vi "Get First 429 Tx Channel.vi"(8 "error in (no error)":errorcluster, 11 "Card Number":i32=2) -> (0 "error out":errorcluster, 2 "Channel Number":i32=32, 3 "Core Number":i32)   [LabVIEW 2019]
uses:
  <instrlib>/BTICardLib/Private/Initialize By Card Number and Core Number.vi
  <instrlib>/BTICardLib/BTICardLV.lvlib
  <instrlib>/BTI429Lib/BTI429LV.lvlib
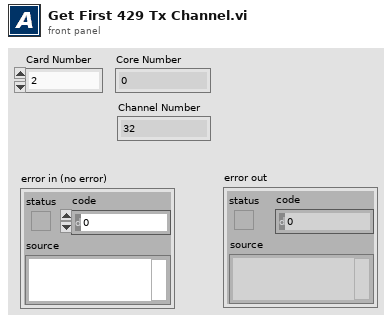
[diagram p1: front panel]
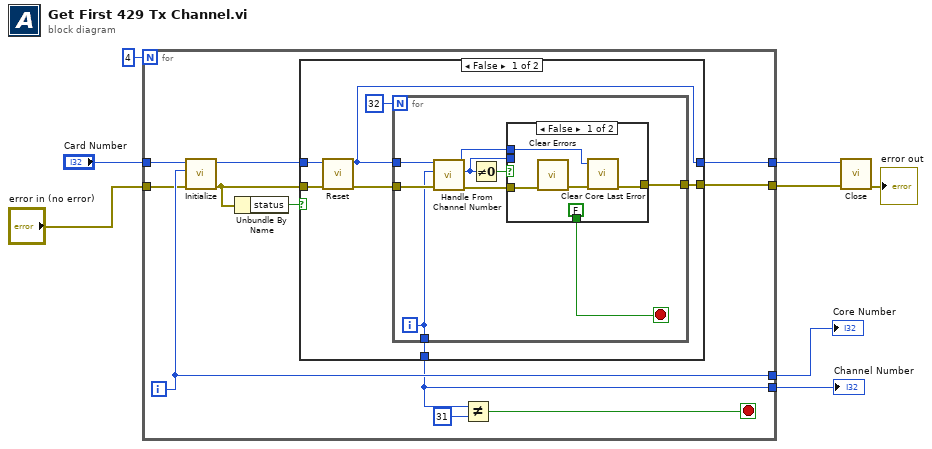
[diagram p0: block diagram]
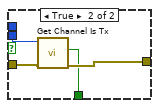
[diagram p2: hidden frame]
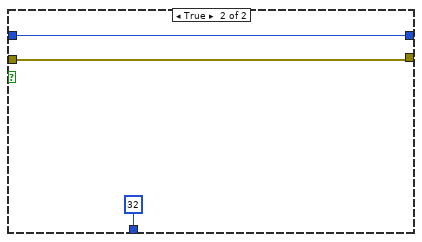
[diagram p3: hidden frame]
diagram:
  n1 = for {
    N: 4 -> [_]
    tunnel: "Card Number" -> [w19]
    tunnel: [w15] -> w6
    tunnel: [w12] -> w5
    tunnel: [w11] -> w4
    tunnel: [w10] -> w3
    tunnel: "error in (no error)" -> [w9]
    i -> [w11]
    stop <- w13 stop-if-true
    n2 = call-poly <instrlib>:"Initialize.vi"("error in (no error)"=w9, "core number"=w11, "card number"=w19) -> ("error out"=w16:errorcluster, "core handle out"=w18:u64)  [unwired: 7 in]
    n3 = Unbundle By Name(w16) -> ("status"=w17:bool)
    n4 = case shown="False" w17 {
      tunnel: w18 -> [w25 w45]
      tunnel: w16 -> [w26 w47]
      tunnel: [w22 w47] -> w15
      tunnel: [w21 32] -> w10
      tunnel: [w20 w45] -> w12
      frame False {
        n5 = call <instrlib>:"Reset.vi"("error in (no error)"=w26, "core handle in"=w25) -> ("error out"=w23:errorcluster, "core handle out"=w20:u64)  [unwired: 8 in]
        n6 = for {
          N: 32 -> [_]
          tunnel: w23 -> [w35]
          tunnel: w20 -> [w34]
          tunnel: [w31] -> w22
          tunnel: [w29] -> w21
          i -> [w29]
          stop <- w30 stop-if-true
          n7 = call <instrlib>:"Handle From Channel Number.vi"("error in (no error)"=w35, "channel number"=w29, "core handle in"=w34) -> ("error out"=w32:errorcluster, "channel handle out"=w28:u64, "core handle out"=w27:u64)  [unwired: 6 in]
          n8 = Not Equal To 0?(x=w28) -> (x != 0?=w33:bool)
          n9 = case shown="False" w33 {
            tunnel: w32 -> [w39 w44]
            tunnel: [w38 w43] -> w31
            tunnel: [FALSE ("channel is receive?") w41] -> w30
            tunnel: w28 -> [_ w42]
            tunnel: w27 -> [w36 _]
            frame False {
              n10 = call <vilib>:"Clear Errors.vi"("error in (no error)"=w39) -> ("error out"=w37:errorcluster)  [unwired: 5 in, 1 out]
              n11 = call <instrlib>:"Clear Core Last Error.vi"("error in (no error)"=w37, "handle in"=w36) -> ("error out"=w38:errorcluster)  [unwired: 8 in, 1 out]
            }
            frame True {
              n12 = call <instrlib>:"Get Channel Is Tx.vi"("error in (no error)"=w44, "channel handle in"=w42) -> ("error out"=w43:errorcluster, "channel is transmit?"=w41:bool)  [unwired: 7 in, 1 out]
            }
          }
        }
      }
      frame True {
      }
    }
    n13 = Not Equal?(x=w10, y=31) -> (x != y?=w13:bool)
  }
  "Core Number" <- w4
  "Channel Number" <- w3
  n14 = call <instrlib>:"Close.vi"("error in (no error)"=w6, "core handle in"=w5) -> ("error out"=→"error out":errorcluster)  [unwired: 8 in, 1 out]
